vi "Self.vi"(9 "Is Priority":bool, 10 "Msg":refnum<class "Msg.lvclass">, 11 "Base Actor in":refnum<class "Base Actor.lvclass">) -> (3 "Base Actor out":refnum<class "Base Actor.lvclass">)   [LabVIEW 2020, in "jettl.lvlib" / "Actor.lvlib" / "Base Actor.lvclass"]
uses:
  Base Actor.lvclass
  Msg/Msg.lvclass
  Relation.ctl
  Actor.lvlib
  Error/Error.lvlib
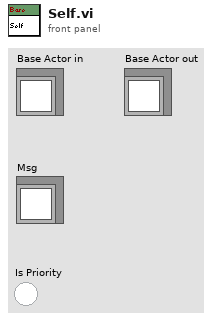
[diagram p1: front panel]
types:
  T1 = typedef "jettl.lvlib/Actor.lvlib/Attributes.ctl" = cluster{"Alias":string, "Address":refnum<user-event>, "Register":refnum<event-registration>, "Implemented Msgs":T2, "Path":path}
  T2 = typedef "jettl.lvlib/Actor.lvlib/Implemented Msgs.ctl" = set{refnum<class "Msg.lvclass">}
  T3 = typedef "jettl.lvlib/Actor.lvlib/Relation.ctl" = enum16{"Self", "Creator", "Created"}
  T4 = typedef "jettl.lvlib/Actor.lvlib/Error Info.ctl" = cluster{"Is Framework Error":bool, "Error":errorcluster}
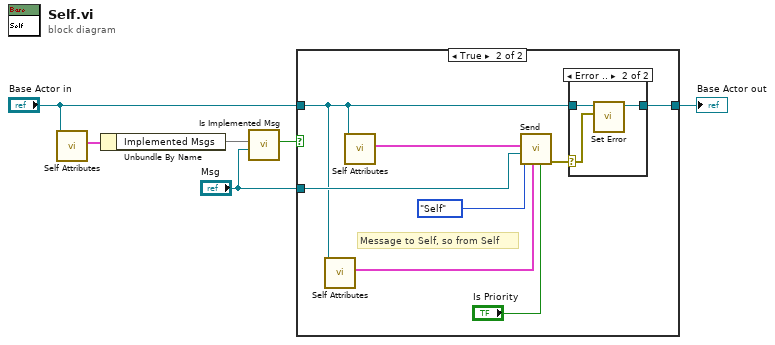
[diagram p0: block diagram]
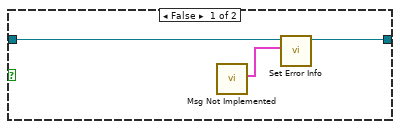
[diagram p2: hidden frame]
diagram:
  n1 = call-dynamic "Self Attributes.vi"("Base Actor in"="Base Actor in") -> ("Self Attributes"=w1:T1)  [unwired: 10 in]
  n2 = Unbundle By Name(w1) -> ("Implemented Msgs"=w5:T2)
  n3 = call "Is Implemented Msg.vi"("Msg"="Msg", "Implemented Msgs"=w5) -> ("Is Implemented Msg"=w4:bool)  [unwired: 9 in]
  n4 = case shown="True" w4 {
    tunnel: [w8 w17] -> w6
    tunnel: "Base Actor in" -> [w9 w15]
    tunnel: "Msg" -> [_ w16]
    frame False {
      n5 = call "Msg Not Implemented.vi"() -> ("Error Info"=w7:T4)  [unwired: 11 in]
      n6 = call "Set Error Info.vi"("Error Info"=w7, "Base Actor in"=w9) -> ("Base Actor out"=w8:refnum<class "Base Actor.lvclass">)  [unwired: 9 in]
    }
    frame True {
      # "Message to Self, so from Self"
      n7 = call-dynamic "Self Attributes.vi"("Base Actor in"=w15) -> ("Self Attributes"=w11:T1)  [unwired: 10 in]
      n8 = call-dynamic "Self Attributes.vi"("Base Actor in"=w15) -> ("Self Attributes"=w13:T1)  [unwired: 10 in]
      n9 = call "Send.vi"("Is Priority"="Is Priority", "Self Attributes"=w11, "Relation"=Relation."Self", "Msg"=w16, "Attributes"=w13) -> ("Error Out"=w14:errorcluster)  [unwired: 6 in]
      n10 = case shown="Error .." w14 {
        selector: w14 -> [_ w19]
        tunnel: [w18 w21] -> w17
        tunnel: w15 -> [w18 w20]
        frame No Error {
        }
        frame Error {
          n11 = call-dynamic "Set Error.vi"("Error"=w19, "Base Actor in"=w20) -> ("Base Actor out"=w21:refnum<class "Base Actor.lvclass">)  [unwired: 9 in]
        }
      }
    }
  }
  "Base Actor out" <- w6
